vi "perform_checks_after_BCK_move.vi"(2 "tour in progress":T1[](array[typedef]), 3 "chessboard":T2[][](array[typedef])) -> (0 "square_to_move_forward_to":T1, 1 "next action":T4)   [LabVIEW 2020, in "core.lvlib"]
uses:
  core.lvlib
  action.ctl
  core_data/chess_square.ctl
  core_data/neighbour_square.ctl
  core_data/chessboard_index.ctl
  pause (global variable).vi
  get all unexplored neighbours.vi
  core_data/core_data.lvlib
panel:
  # "Development\ncontrols/indicators useful for development and testing, but which are not outputs of the VI"
  # "Input\nInputs to the VI"
  # "Output\nOutputs of the VI"
  # "Description\n\nBlank VI with error handling case. \n\nSummarize the use of this VI in this space."
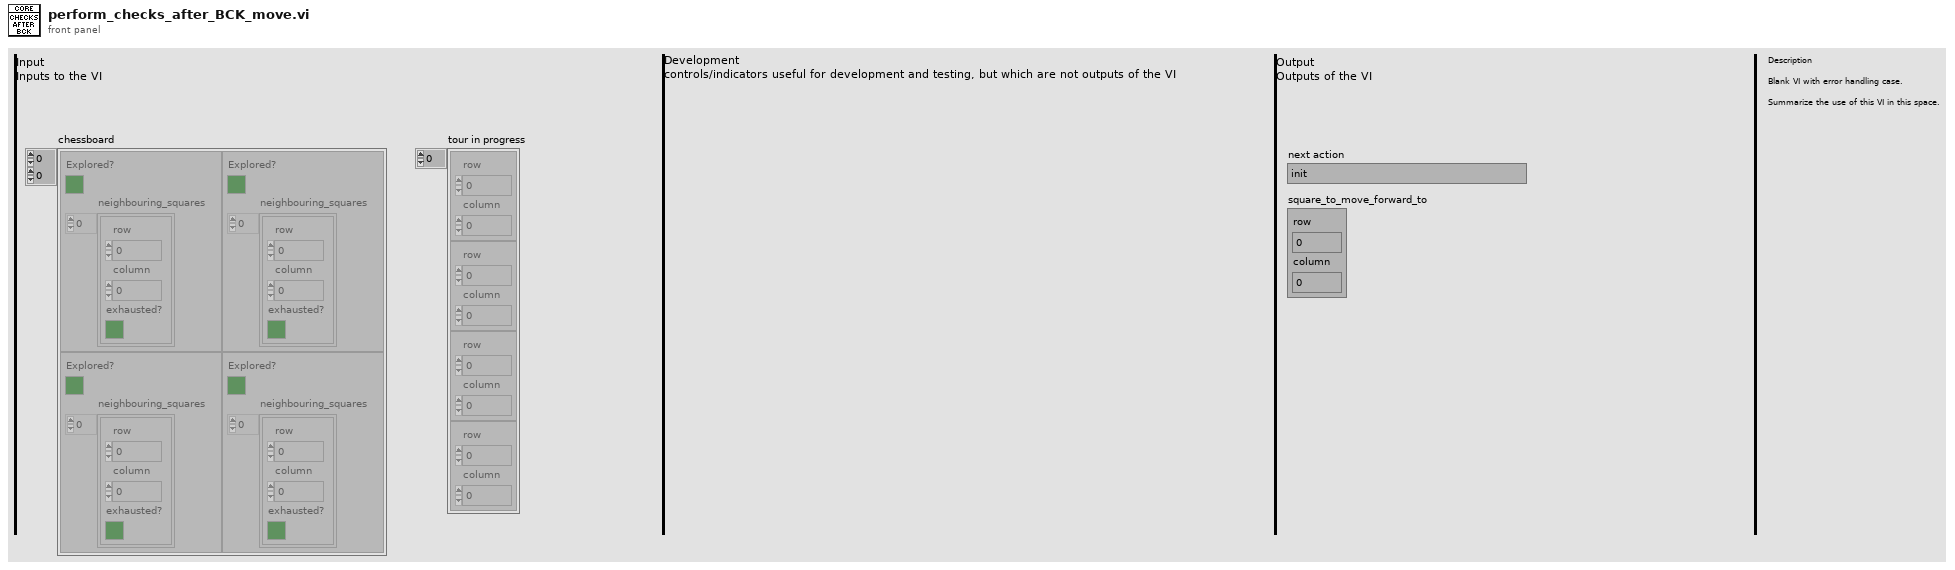
[diagram p1: front panel]
types:
  T1 = typedef "core.lvlib/core_data.lvlib/chessboard_index.ctl" = cluster{"row":u8, "column":u8}
  T2 = typedef "core.lvlib/core_data.lvlib/chess_square.ctl" = cluster{"Explored?":bool, "neighbouring_squares":T3[]}
  T3 = typedef "core.lvlib/core_data.lvlib/neighbour_square.ctl" = cluster{"row":u8, "column":u8, "exhausted?":bool}
  T4 = typedef "core.lvlib/action.ctl" = enum16{"init", "move_forward", "move_backward", "complete_tour", "exit", "be idle (do nothing)"}
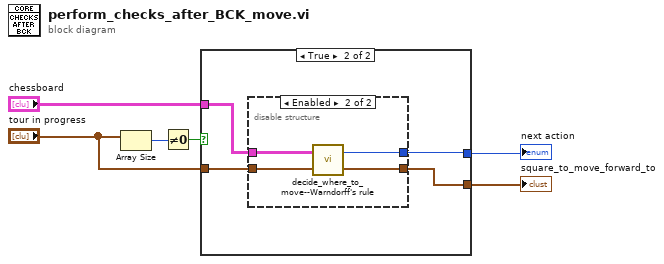
[diagram p0: block diagram]
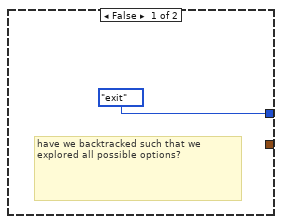
[diagram p2: hidden frame]
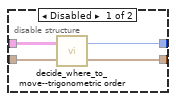
[diagram p3: hidden frame]
diagram:
  n1 = Array Size(array="tour in progress") -> (size(s)=w6:i32)
  n2 = Not Equal To 0?(x=w6) -> (x != 0?=w5:bool)
  n3 = case shown="True" w5 {
    tunnel: [action."exit" ("action") w11] -> w4
    tunnel: "chessboard" -> [_ w10]
    tunnel: "tour in progress" -> [_ w9]
    tunnel: [_ w8] -> w1
    frame False {
      # "have we backtracked such that we explored all possible options?"
    }
    frame True {
      n4 = disable-structure shown="Enabled" {
        disable-tunnel: [w15 w17] -> w11
        disable-tunnel: w10 -> [w14 w18]
        disable-tunnel: w9 -> [w13 w19]
        disable-tunnel: [w12 w16] -> w8
        frame Disabled {
          n5 = call "decide_where_to_move--trigonometric order.vi"("tour_in_progress"=w13, "chessboard"=w14) -> ("square_to_move_forward_to"=w12:T1, "action"=w15:T4)
        }
        frame Enabled {
          n6 = call "decide_where_to_move--Warndorff's rule.vi"("tour_in_progress"=w19, "chessboard"=w18) -> ("square_to_move_forward_to"=w16:T1, "action"=w17:T4)
        }
      }
    }
  }
  "next action" <- w4
  "square_to_move_forward_to" <- w1
